vi "Get Custom Device Name.vi"(8 "error in":errorcluster, 11 "XML Node":refnum<k20>) -> (0 "error out":errorcluster, 2 "Custom Device Name":string, 3 "XML Node out":refnum<k20>)   [LabVIEW 2024, in "Config File Parser.lvlib" / "Custom Device Config.lvclass"]
uses:
  Custom Device Config.lvclass
  <vilib>/xml/Close Reference(Node).vi
  Custom Device Config.lvclass/Custom Device Config.ctl
  <resource>/objmgr/DOMUserDefRef.rc
  <vilib>/xml/NI_XML.lvlib
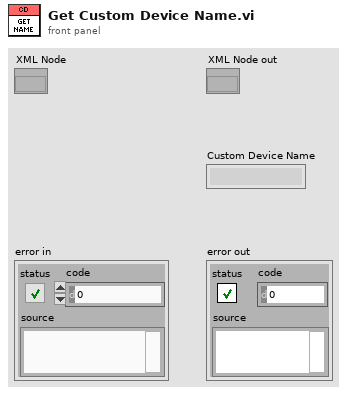
[diagram p1: front panel]
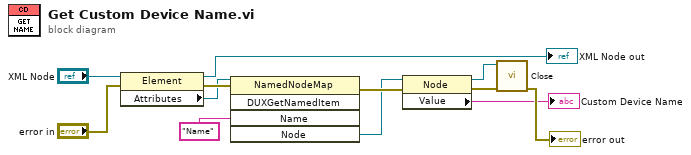
[diagram p0: block diagram]
diagram:
  n1 = property on="Property Node" class="Element"(reference="XML Node", error in="error in") -> (reference out=→"XML Node out":refnum<k20>, error out=w12:errorcluster, "Attributes"=w6:refnum<k20>)
  n2 = invoke on="Invoke Node" class="NamedNodeMap" method="DUXGetNamedItem"(reference=w6, error in=w12, "Name"="Name") -> (error out=w10:errorcluster, "Node"=w4:refnum<k20>)  [unwired: 2 in, 3 out]
  n3 = property on="Property Node" class="Node"(reference=w4, error in=w10) -> (reference out=w2:refnum<k20>, error out=w9:errorcluster, "Value"=→"Custom Device Name":string)
  n4 = call-poly <vilib>:"Close.vi"("error in (no error)"=w9, "node"=w2) -> ("error out"=→"error out":errorcluster)  [unwired: 7 in]
